vi "Get.vi"(11 "Text in":refnum<class "Text.lvclass">) -> (2 "Value":string)   [LabVIEW 2022 SP3, in "Conditum.lvlib" / "Columns.lvlib" / "Text.lvclass"]
uses:
  Text.lvclass
  Text.lvclass/Text.ctl
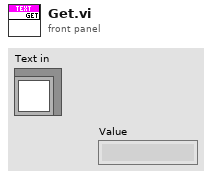
[diagram p1: front panel]
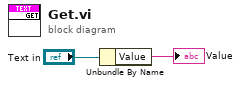
[diagram p0: block diagram]
diagram:
  n1 = Unbundle By Name("Text in") -> ("Value"=→"Value":string)
